vi "task_Keybut_ActiveCmd.vi"(8 "error in (no error)":errorcluster, 10 "update":bool, 11 "New AppCmd":T1) -> (0 "error out":errorcluster, 3 "AppCmd":T1)   [LabVIEW 2015]
uses:
  UsrDefine/imt_app_cmd.ctl
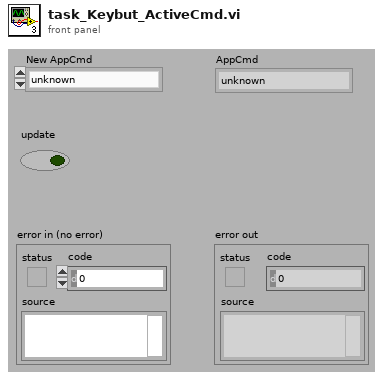
[diagram p1: front panel]
types:
  T1 = typedef "imt_app_cmd.ctl" = enum16{"unknown", "configHardware", "configDevice", "updateFirmware", "usb_scope"}
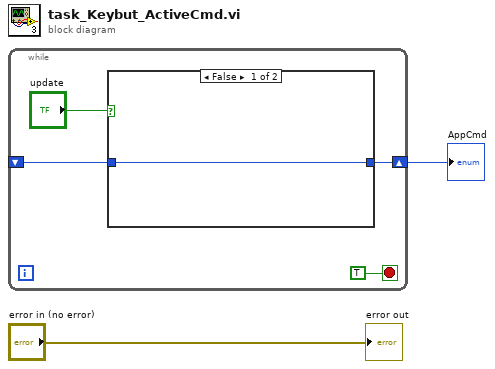
[diagram p0: block diagram]
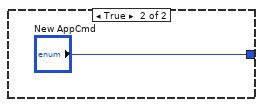
[diagram p2: hidden frame]
diagram:
  n1 = while {
    shift-right: [w4] -> w1
    shift-left: _ -> [w3]
    stop <- TRUE stop-if-true
    n2 = case shown="False" "update" {
      tunnel: [w7 "New AppCmd"] -> w4
      tunnel: w3 -> [w7 _]
      frame False {
      }
      frame True {
      }
    }
  }
  "AppCmd" <- w1
  "error out" <- "error in (no error)"
